vi "ScaleTargetVector.vi"(10 "Target Vector Norm":T2) -> (2 "Target Vector":T1)   [LabVIEW 2018]
uses:
  Util/Math/Vector/Vector3D.ctl
  Util/Math/Vector/Vector2D.ctl
  Util/Math/Vector/Vector3DtoVector2D_XY.vi
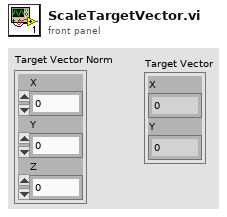
[diagram p1: front panel]
types:
  T1 = typedef "Vector2D.ctl" = cluster{"X":dbl, "Y":dbl}
  T2 = typedef "Vector3D.ctl" = cluster{"X":dbl, "Y":dbl, "Z":dbl}
  T3 = typedef "Constants.ctl" = cluster{"WheelSensorCountPerRevolution":dbl, "WheelDiameter":dbl, "WheelInchPerSensorUnit":dbl, "kSystemS(V)":dbl, "MaxVelocityRawUnits":dbl, "MaxAccelRawUnits":dbl, "PowerMMGains":cluster{"P Gain":dbl, "I Gain":dbl, "D Gain":dbl, "F Gain":dbl, "I Zone":dbl, "Min Output":dbl, "Max Output":dbl}, "SwerveModuleTopHeight":dbl, "CameraMountLenseHeight":dbl, "CameraLenseHeight":dbl, "CameraMountPitch":dbl, "CameraMountYaw":dbl, "HatchTargetHeight":dbl, "RocketPortTargetHeight":dbl, "Camera Lense Rel Pos":T2}
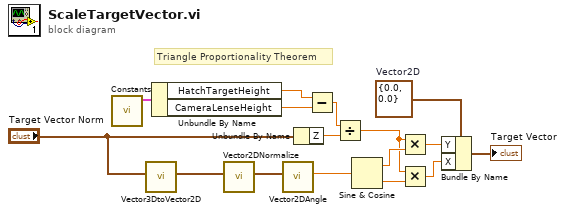
[diagram p0: block diagram]
diagram:
  w3 = T1 {"X"=0.0, "Y"=0.0}  # Vector2D
  # "Triangle Proportionality Theorem"
  n1 = call "Constants.vi"() -> ("Constants"=w16:T3)  [unwired: 11 in]
  n2 = call-poly "Vector3DtoVector2D.vi"("Vector3D"="Target Vector Norm") -> ("Vector2D"=w10:T1)  [unwired: 10 in]
  n3 = Unbundle By Name(w16) -> ("HatchTargetHeight"=w12:dbl, "CameraLenseHeight"=w14:dbl)
  n4 = call "Vector2DNormalize.vi"("Vector"=w10) -> ("Normalized Vector"=w9:T1)  [unwired: 10 in]
  n5 = call "Vector2DAngle.vi"("Vector2D"=w9) -> ("Angle"=w8:dbl)  [unwired: 10 in]
  n6 = Unbundle By Name("Target Vector Norm") -> ("Z"=w13:dbl)
  n7 = Subtract(x=w12, y=w14) -> (x-y=w15:dbl)
  n8 = Divide(x=w15, y=w13) -> (x/y=w5:dbl)
  n9 = Sine & Cosine(0:w8) -> (1:w7:dbl, 2:w6:dbl)
  n10 = Multiply(x=w5, y=w7) -> (x*y=w4:dbl)
  n11 = Multiply(x=w5, y=w6) -> (x*y=w2:dbl)
  n12 = Bundle By Name(cluster=w3, "Y"=w4, "X"=w2) -> (→"Target Vector":T1)
